vi "Meas Result Make Cplx Unc Bars to Graph.vi"(3 "unc y":dbl[](array[numeric]), 4 "y":dbl[](array[numeric]), 5 "unc x":dbl[](array[numeric]), 6 "x":dbl[](array[numeric])) -> (0 "trace":cluster{dbl[], dbl[]}, 1 "y out":dbl[](array[numeric]), 2 "x out":dbl[](array[numeric]))   [LabVIEW 2020]
doc: "Simulates x-y uncertainty bars to graph by inserting vertical and horizontal offsets to vector of graph values."
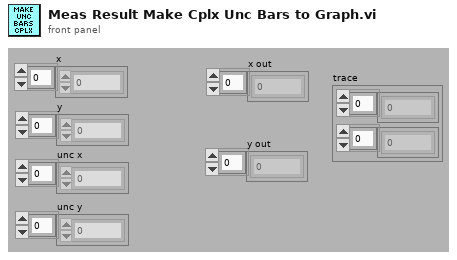
[diagram p1: front panel]
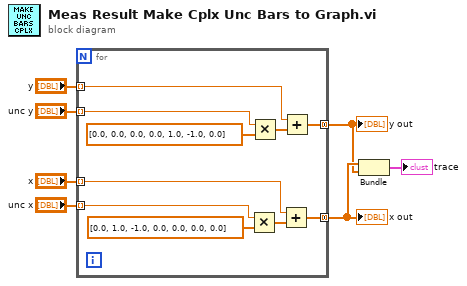
[diagram p0: block diagram]
diagram:
  n1 = for {
    tunnel: "y" -> [w12] mode=indexing
    tunnel: "unc x" -> [w14] mode=indexing
    tunnel: [w9] -> w4 mode=concatenating
    tunnel: [w8] -> w5 mode=concatenating
    tunnel: "unc y" -> [w16] mode=indexing
    tunnel: "x" -> [w10] mode=indexing
    n2 = Multiply(x=w14, y=dbl[] [0.0, 1.0, -1.0, 0.0, 0.0, 0.0, 0.0]) -> (x*y=w11:dbl[])
    n3 = Multiply(x=w16, y=dbl[] [0.0, 0.0, 0.0, 0.0, 1.0, -1.0, 0.0]) -> (x*y=w13:dbl[])
    n4 = Add(x=w10, y=w11) -> (x+y=w8:dbl[])
    n5 = Add(x=w12, y=w13) -> (x+y=w9:dbl[])
  }
  "x out" <- w5
  "y out" <- w4
  n6 = Bundle(w5, w4) -> (→"trace":cluster{dbl[], dbl[]})  [unwired: 1 in]
